vi "Join.vi"(6 "delimiter":string, 11 "Array":string[](array[string])) -> (3 "Joined Result":string)   [LabVIEW 2009]
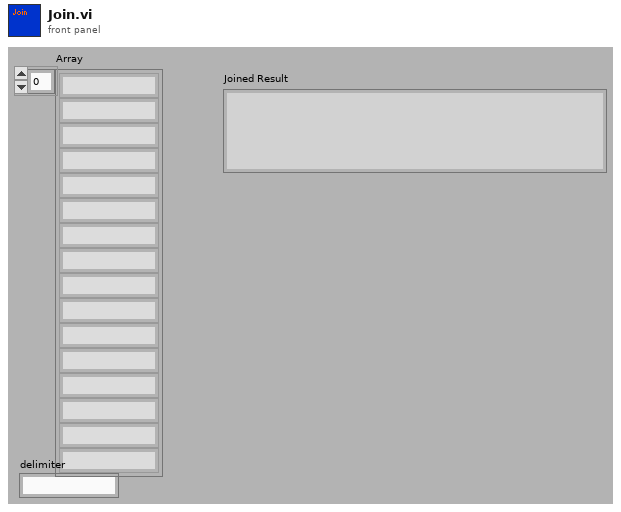
[diagram p1: front panel]
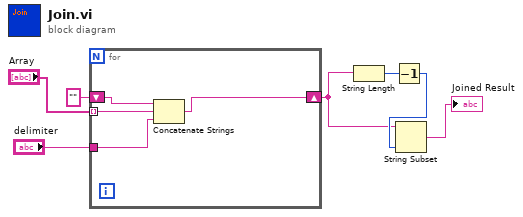
[diagram p0: block diagram]
diagram:
  n1 = for {
    tunnel: "Array" -> [w11] mode=indexing
    shift-right: [w9] -> w3
    shift-left: "" -> [w10]
    tunnel: "delimiter" -> [w8]
    n2 = Concatenate Strings(w10, w11, w8) -> (w9:string)
  }
  n3 = String Length(string=w3) -> (length=w5:i32)
  n4 = Decrement(x=w5) -> (x-1=w4:i32)
  n5 = String Subset(string=w3, length (rest)=w4) -> (substring=→"Joined Result":string)  [unwired: 1 out]
